vi "Burn In Test.vi"(8 "error in (no error)":errorcluster, 9 "max time milliseconds (10 seconds)":i32=10000, 10 "script name":string, 11 "Semiconductor Module Context":T1) -> (0 "error out":errorcluster)   [LabVIEW 2013]
uses:
  <vilib>/NI_TestStand_SemiconductorModule/NI_TestStand_Semiconductor_Module.lvlibp/PinMap/General/SemiconductorModuleContext.ctl
  <vilib>/NI_TestStand_SemiconductorModule/NI_TestStand_Semiconductor_Module.lvlibp
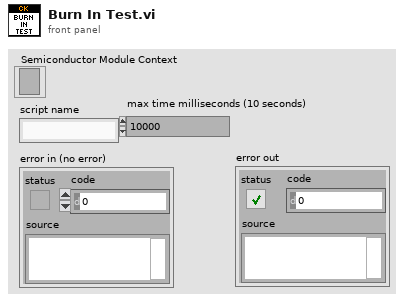
[diagram p1: front panel]
types:
  T1 = typedef "NI_TestStand_Semiconductor_Module.lvlibp/SemiconductorModuleContext.ctl" = refnum<k7>
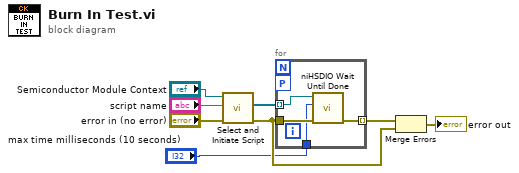
[diagram p0: block diagram]
diagram:
  n1 = call "Select and Initiate Script.vi"("error in (no error)"="error in (no error)", "script name"="script name", "Semiconductor Module Context"="Semiconductor Module Context") -> ("error out"=w3:errorcluster, "HSDIO GEN Sessions Out"=w6:refnum<k15>[])  [unwired: 6 in, 1 out]
  n2 = for {
    tunnel: w3 -> [w12]
    tunnel: w6 -> [w11] mode=indexing
    tunnel: [w10] -> w5 mode=indexing
    workers-P: _ -> [_]
    tunnel: "max time milliseconds (10 seconds)" -> [w9]
    n3 = call <instrlib>:"niHSDIO Wait Until Done.vi"("error in (no error)"=w12, "max time milliseconds (10 seconds)"=w9, "instrument handle"=w11) -> ("error out"=w10:errorcluster)  [unwired: 7 in, 1 out]
  }
  n4 = Merge Errors(w5, w3) -> (→"error out":errorcluster)
